vi "Write Instrument.vi"(8 "error in (no error)":errorcluster, 10 "Instrument in":refnum<class "Instrument Driver.lvclass">, 11 "Actor in":refnum<class "Actor.lvclass">) -> (0 "error out":errorcluster, 3 "Instrument Owner out":refnum<class "Instrument Owner.lvclass">)   [LabVIEW 2020, in "Instrument Handler.lvlib" / "Instrument Owner.lvclass"]
doc: "This VI exposes the Write Instrument to the Community Scope."
uses:
  Instrument Owner.lvclass
  PPL/HDH.Actor Framework.Core.Actor.lvlibp/1abvi3w/vi.lib/ActorFramework/Actor/Actor.lvclass
  PPL/HDH.Actor Framework.Core.Instrument Driver.lvlibp/Instrument Driver/Instrument Driver.lvclass
  Instrument Sequencer/Instrument Sequencer.lvclass
  Instrument Sequencer/Instrument Sequencer.lvclass/Instrument Sequencer.ctl
  PPL/HDH.Actor Framework.Core.Sequencer.lvlibp/Sequencer/Sequencer.lvclass
  C:/Current projects/WS/PPL/HDH.Actor Framework.Core.Sequencer.lvlibp/Sequencer/Sequencer.lvclass
  C:/Current projects/WS/PPL/HDH.Actor Framework.Core.Sequencer.lvlibp/Sequencer Core/Sequencer Core.lvclass
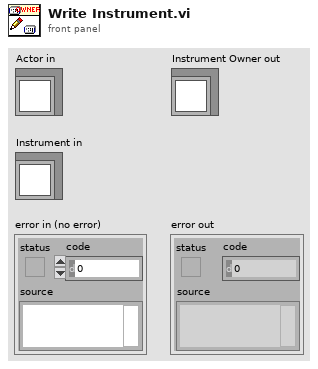
[diagram p1: front panel]
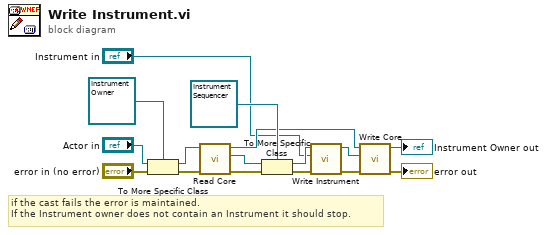
[diagram p0: block diagram]
diagram:
  # "if the cast fails the error is maintained. \nIf the Instrument owner does not contain an Instrument it should stop."
  n1 = To More Specific Class(target class=refnum<class "Instrument Owner.lvclass"> refnum ("Instrument Handler.lvlib:Instrument Owner.lvclass"), reference="Actor in", error in="error in (no error)") -> (specific class reference=w2:refnum<class "Instrument Owner.lvclass">, error out=w4:errorcluster)
  n2 = call "Read Core.vi"("error in (no error)"=w4, "Sequencer in"=w2) -> ("error out"=w9:errorcluster, "Core"=w15:refnum<class "Sequencer Core.lvclass">, "Sequencer out"=w12:refnum<class "Instrument Owner.lvclass">)  [unwired: 7 in]
  n3 = To More Specific Class(target class=refnum<class "Instrument Sequencer.lvclass"> refnum ("Instrument Handler.lvlib:Instrument Sequencer.lvclass"), reference=w15, error in=w9) -> (specific class reference=w13:refnum<class "Instrument Sequencer.lvclass">, error out=w8:errorcluster)
  n4 = call "Write Instrument.vi"("error in (no error)"=w8, "Instrument Driver"="Instrument in", "Instrument Sequencer in"=w13) -> ("error out"=w7:errorcluster, "Instrument Sequencer out"=w11:refnum<class "Instrument Sequencer.lvclass">)  [unwired: 7 in]
  n5 = call "Write Core.vi"("error in (no error)"=w7, "Core in"=w11, "Sequencer in"=w12) -> ("error out"=→"error out":errorcluster, "Sequencer out"=→"Instrument Owner out":refnum<class "Instrument Owner.lvclass">)  [unwired: 7 in]
